vi "Exit Windows.vi"(8 "command line argument (N/A)":string, 9 "DOS command line (N/A)":string, 10 "show prompt? (T)":bool=TRUE, 11 "exit windows function (1)":u32(ring)=1 items=["Log off", "Shut Down", "Exit Windows and Reboot"]) -> (0 "error out":errorcluster)   [LabVIEW 2023, in "Winevent.lvlib"]
doc: "This VI allows you to exit windows in various ways.\nexit windows function\n0: Log off\n1: Shut Down\n2: Exit Windows and reboot the computer"
uses:
  Winevent.lvlib
  user32.dll
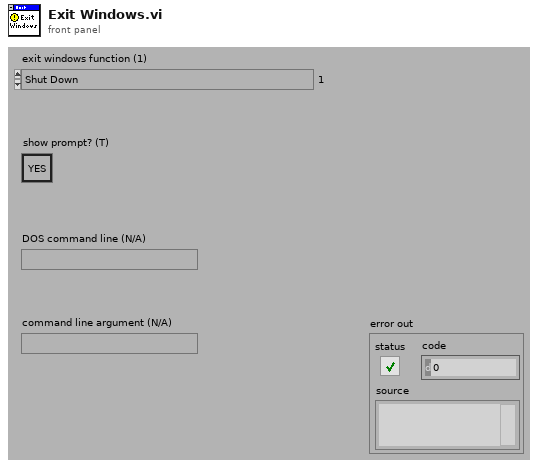
[diagram p1: front panel]
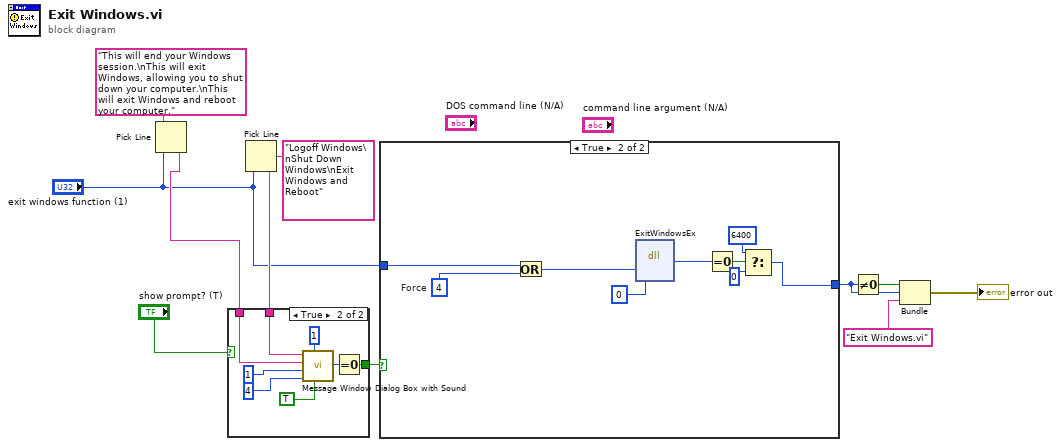
[diagram p0: block diagram]
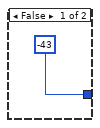
[diagram p2: hidden frame]
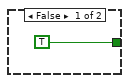
[diagram p3: hidden frame]
diagram:
  n1 = Pick Line(multi-line string="This will end your Windows session.\nThis will exit Windows, allowing you to shut down your computer.\nThis will exit Windows and reboot your computer.", line index="exit windows function (1)") -> (output string=w6:string)  [unwired: 1 out]
  n2 = Pick Line(multi-line string="Logoff Windows\nShut Down Windows\nExit Windows and Reboot", line index="exit windows function (1)") -> (output string=w7:string)  [unwired: 1 out]
  n3 = case shown="True" "show prompt? (T)" {
    tunnel: [TRUE w19] -> w10
    tunnel: w7 -> [_ w14]
    tunnel: w6 -> [_ w13]
    frame False {
    }
    frame True {
      n4 = call "Message Window Dialog Box with Sound.vi"("sound? (F)"=TRUE, "modality (0)"=1, "icon (0:None)"=4, "buttons (0:OK)"=1, "message (\"\")"=w13, "window title (\"\")"=w14) -> ("button pressed"=w18:i32)
      n5 = Equal To 0?(x=w18) -> (x = 0?=w19:bool)
    }
  }
  n6 = case shown="True" w10 {
    tunnel: [-43 w30] -> w4
    tunnel: "exit windows function (1)" -> [_ w24]
    frame False {
    }
    frame True {
      w23 = u32 4  # Force
      n7 = Or(x=w24, y=w23) -> (x .or. y?=w22:u32)
      n8 = dll-call lib="user32.dll" fn="ExitWindowsEx" label="ExitWindows"("returnCode"=w22, "reserved (set to zero)"=u32 0) -> (w26:i32)  [unwired: 5 in, 2 out]
      n9 = Equal To 0?(x=w26) -> (x = 0?=w27:bool)
      n10 = Select(t=6400, s=w27, f=0) -> (s? t:f=w30:i32)
    }
  }
  n11 = Not Equal To 0?(x=w4) -> (x != 0?=w5:bool)
  n12 = Bundle(w5, w4, "Exit Windows.vi") -> (→"error out":errorcluster)  [unwired: 1 out]
